vi "Set_Parameter.vi"(8 "error in (no error)":errorcluster, 10 "DeviceConfig":T1, 11 "Avantes in":refnum<class "Avantes.lvclass">) -> (0 "error out":errorcluster, 3 "Avantes out":refnum<class "Avantes.lvclass">)   [LabVIEW 2020, in "Avantes.lvclass"]
uses:
  <instrlib>/Classes/CCD/Avantes/Avantes.lvclass
  <instrlib>/Devices/Avantes/clusterdef.ctl
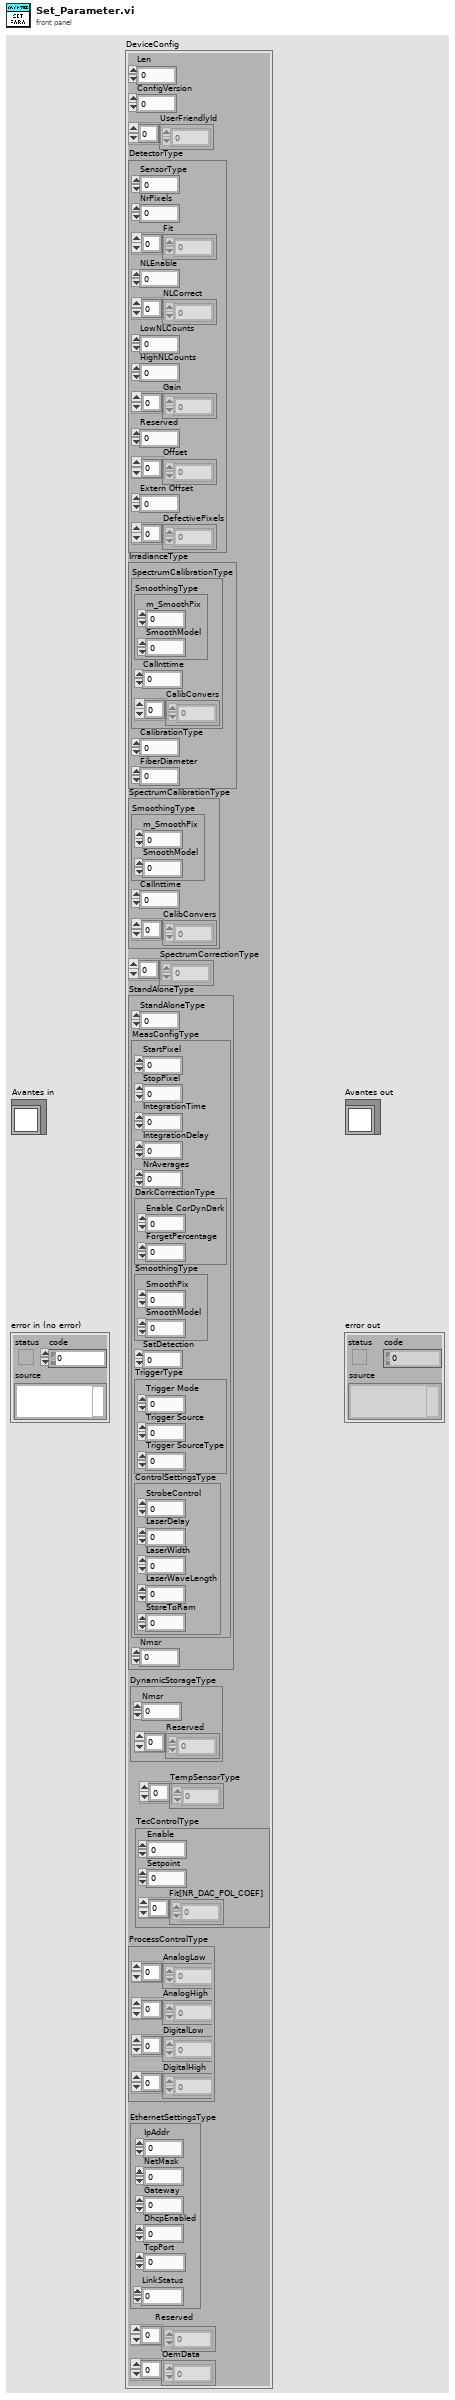
[diagram p1: front panel]
types:
  T1 = typedef "clusterdef.ctl" = cluster{"Len":u16, "ConfigVersion":u16, "UserFriendlyId":u8[], "DetectorType":cluster{"SensorType":u8, "NrPixels":u16, "Fit":sgl[], "NLEnable":u8, "NLCorrect":dbl[], "LowNLCounts":dbl, "HighNLCounts":dbl, "Gain":sgl[], "Reserved":sgl, "Offset":sgl[], "Extern Offset":sgl, "DefectivePixels":u16[]}, "IrradianceType":cluster{"SpectrumCalibrationType":cluster{"SmoothingType":cluster{"m_SmoothPix":u16, "SmoothModel":u8}, "CalInttime":sgl, "CalibConvers":sgl[]}, "CalibrationType":u8, "FiberDiameter":i32}, "SpectrumCalibrationType":cluster{"SmoothingType":cluster{"m_SmoothPix":u16, "SmoothModel":u8}, "CalInttime":sgl, "CalibConvers":sgl[]}, "SpectrumCorrectionType":sgl[], "StandAloneType":cluster{"StandAloneType":u8, "MeasConfigType":cluster{"StartPixel":u16, "StopPixel":u16, "IntegrationTime":sgl, "IntegrationDelay":u32, "NrAverages":u32, "DarkCorrectionType":cluster{"Enable CorDynDark":u8, "ForgetPercentage":u8}, "SmoothingType":cluster{"SmoothPix":u16, "SmoothModel":u8}, "SatDetection":u8, "TriggerType":cluster{"Trigger Mode":u8, "Trigger Source":u8, "Trigger SourceType":u8}, "ControlSettingsType":cluster{"StrobeControl":u16, "LaserDelay":u32, "LaserWidth":u32, "LaserWaveLength":sgl, "StoreToRam":u16}}, "Nmsr":i16}, "DynamicStorageType":cluster{"Nmsr":i32, "Reserved":u8[]}, "TempSensorType":sgl[], "TecControlType":cluster{"Enable":u8, "Setpoint":sgl, "Fit[NR_DAC_POL_COEF]":sgl[]}, "ProcessControlType":cluster{"AnalogLow":sgl[], "AnalogHigh":sgl[], "DigitalLow":sgl[], "DigitalHigh":sgl[]}, "EthernetSettingsType":cluster{"IpAddr":u32, "NetMask":u32, "Gateway":u32, "DhcpEnabled":u8, "TcpPort":u16, "LinkStatus":u8}, "Reserved":u8[], "OemData":u8[]}
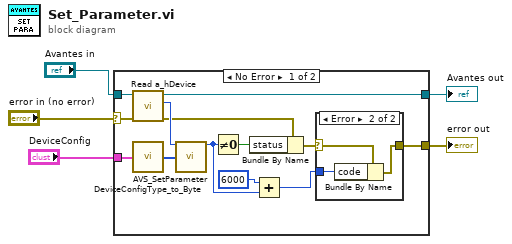
[diagram p0: block diagram]
diagram:
  n1 = case shown="No Error" "error in (no error)" {
    selector: "error in (no error)" -> [w17 w24]
    tunnel: [w7 w24] -> w4
    tunnel: [w13 w23] -> w2
    tunnel: "Avantes in" -> [w18 w23]
    tunnel: "DeviceConfig" -> [w14 _]
    frame No Error {
      n2 = call-dynamic "Read a_hDevice.vi"("error in (no error)"=w17, "Avantes in"=w18) -> ("error out"=w12:errorcluster, "a_hDevice"=w15:i32, "Avantes out"=w13:refnum<class "Avantes.lvclass">)  [unwired: 7 in]
      n3 = call <instrlib>:"DeviceConfigType_to_Byte.vi"("DeviceConfig"=w14) -> ("Byte Array"=w16:u8[])  [unwired: 4 in]
      n4 = call <instrlib>:"AVS_SetParameter.vi"("a_hDevice"=w15, "a_pDeviceParm"=w16) -> ("Output Value"=w9:i32)  [unwired: 12 in, 1 out]
      n5 = Not Equal To 0?(x=w9) -> (x != 0?=w11:bool)
      n6 = Bundle By Name(cluster=w12, "status"=w11) -> (w8:errorcluster)
      n7 = Add(x=6000, y=w9) -> (x+y=w6:i32)
      n8 = case shown="Error" w8 {
        selector: w8 -> [w19 w22]
        tunnel: [w19 w20] -> w7
        tunnel: w6 -> [_ w21]
        frame No Error {
        }
        frame Error {
          n9 = Bundle By Name(cluster=w22, "code"=w21) -> (w20:errorcluster)
        }
      }
    }
    frame Error {
    }
  }
  "error out" <- w4
  "Avantes out" <- w2
